vi "calibrate speed.vi"() -> ()   [LabVIEW 2012]
uses:
  <vilib>/DAQmx/configure/timing.llb/DAQmx Timing (Implicit).vi
  <resource>/objmgr/daqmx.rc
panel:
  out "x+y":dbl
  in  "pulse rev":i32
  in  "dist mm":i32
  in  "speed (mm/s)":dbl
  in  "Direction":bool
  out "samples":i32
  in  "error in":errorcluster
  out "mm/s (timed)":dbl
  out "error out":errorcluster
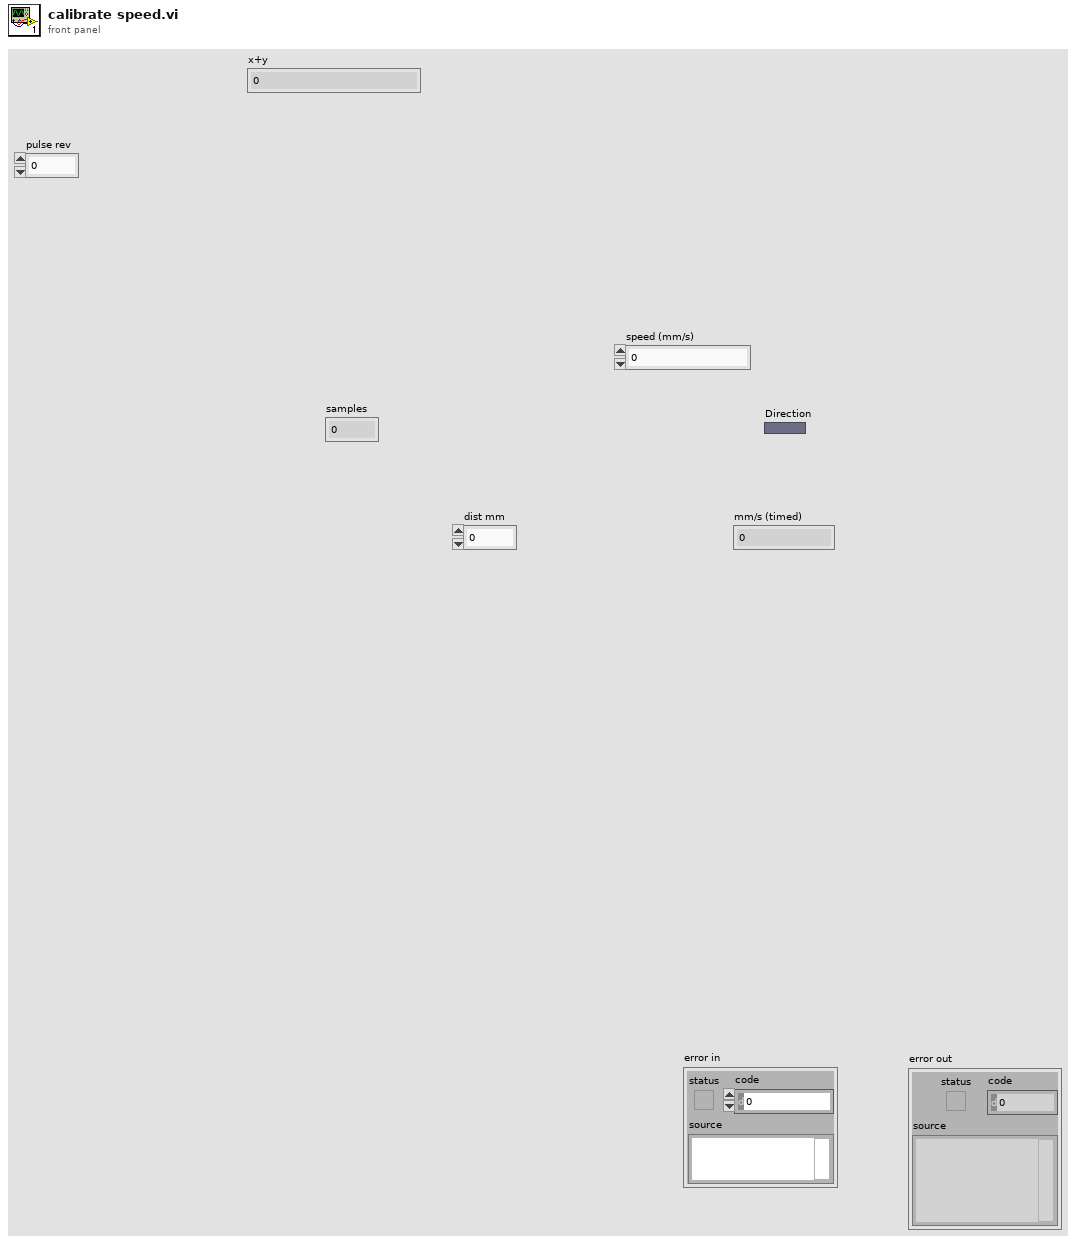
[diagram p1: front panel]
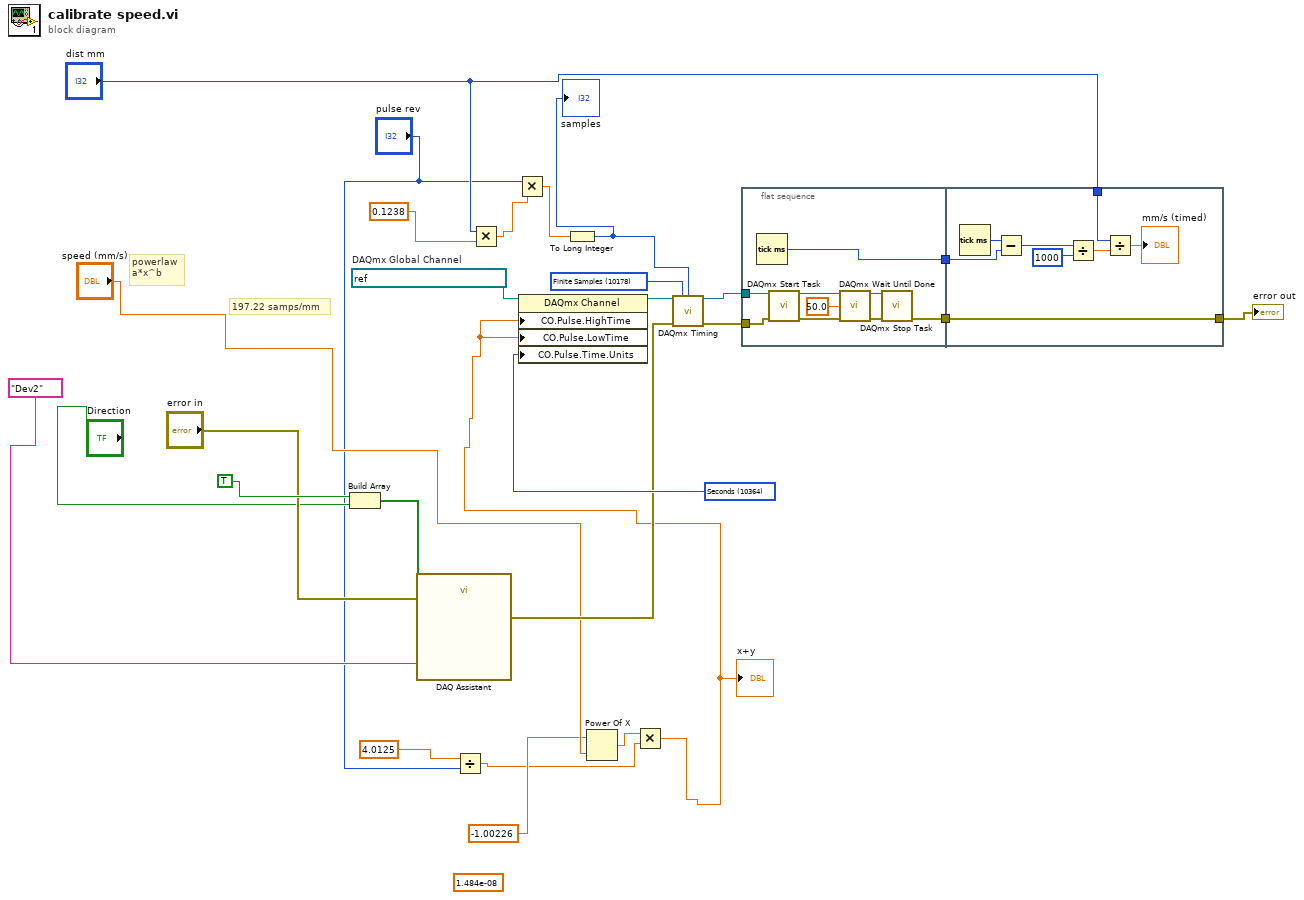
[diagram p0: block diagram]
diagram:
  (unwired) 1.484e-08
  w25 = 10364 items=["Seconds"=10364] ("CO.Pulse.Time.Units")
  w22 = 10178 items=["Finite Samples"=10178, "Continuous Samples"=10123, "Hardware Timed Single Point"=12522] ("sample mode")
  w21 = refnum<k21> "MyPulseOutputChannel"  # DAQmx Global Channel
  # "powerlaw\na*x^b"
  # "197.22 samps/mm"
  n1 = Build Array(TRUE ("element"), "Direction") -> (w20:bool[])
  n2 = call "DAQ Assistant"("data"=w20, "error in"="error in", "device name"=tag "Dev2") -> ("error out"=w16:errorcluster)  [unwired: 15 in, 1 out]
  n3 = Divide(x=4.0125, y="pulse rev") -> (x/y=w1:dbl)
  n4 = Multiply(x="dist mm", y=0.1238) -> (x*y=w9:dbl)
  n5 = Multiply(x="pulse rev", y=w9) -> (x*y=w8:dbl)
  n6 = To Long Integer(number=w8) -> (32bit integer=w14:i32)
  "samples" <- w14
  n7 = Power Of X(1:"speed (mm/s)", 2:-1.00226) -> (0:w5:dbl)
  n8 = Multiply(x=w5, y=w1) -> (x*y=w4:dbl)
  "x+y" <- w4
  n9 = property class="DAQmx Channel"(reference=w21, "CO.Pulse.HighTime"=w4, "CO.Pulse.LowTime"=w4, "CO.Pulse.Time.Units"=w25) -> (reference out=w24:refnum<k21>)  [unwired: 1 in, 1 out]
  n10 = call-poly <vilib>:"DAQmx Timing.vi"("task/channels in"=w24, "sample mode"=w22, "samples per channel"=w14, "error in"=w16) -> ("task out"=w23:refnum<k21>, "error out"=w17:errorcluster)  [unwired: 10 in]
  n11 = flat-sequence {
    tunnel: w23 -> [w34]
    tunnel: [w30] -> w27
    tunnel: [w29] -> w26
    tunnel: w17 -> [w28]
    tunnel: w27 -> [w44]
    tunnel: "dist mm" -> [w40]
    tunnel: w26 -> [w37]
    tunnel: [w37] -> w18
    frame #0 {
      n12 = Tick Count (ms)() -> (millisecond timer value=w30:u32)
      n13 = call <vilib>:"DAQmx Start Task.vi"("task/channels in"=w34, "error in"=w28) -> ("task out"=w35:refnum<k21>, "error out"=w32:errorcluster)  [unwired: 12 in]
      n14 = call <vilib>:"DAQmx Wait Until Done.vi"("task/channels in"=w35, "timeout (sec)"=50.0, "error in"=w32) -> ("task out"=w33:refnum<k21>, "error out"=w31:errorcluster)  [unwired: 11 in]
      n15 = call <vilib>:"DAQmx Stop Task.vi"("task/channels in"=w33, "error in"=w31) -> ("error out"=w29:errorcluster)  [unwired: 12 in, 1 out]
    }
    frame #1 {
      n16 = Tick Count (ms)() -> (millisecond timer value=w43:u32)
      n17 = Subtract(x=w43, y=w44) -> (x-y=w42:u32)
      n18 = Divide(x=w42, y=u32 1000) -> (x/y=w39:dbl)
      n19 = Divide(x=w40, y=w39) -> (x/y=→"mm/s (timed)":dbl)
    }
  }
  "error out" <- w18
